vi "Add Rx Frames.vi"(8 "error in (no error)":errorcluster, 10 "CAN Frames":T1[](array[typedef]) {"payload" format="%x"; "timestamp" format="%<%.7X\n%x>T"; "type" items=["CAN Data"=0, "CAN Remote"=1, "CAN Bus Error"=2, "CAN 2.0 Data"=8, "CAN FD Data"=16, "CAN FD+BRS Data"=24, "J1939 Data"=192, "Delay"=224, "Log Trigger"=225, "Start Trigger"=226]; "identifier" format="%x"}, 11 "CANBus_Load_Calculator in":refnum<class "CANBus_Load_Calculator.lvclass">) -> (0 "error out":errorcluster, 3 "CANBus_Load_Calculator out":refnum<class "CANBus_Load_Calculator.lvclass">)   [LabVIEW 2018, in "NI-XNET Monitor Engine.lvlib" / "XNET-Bus-Load-Calculator.lvlib" / "CANBus_Load_Calculator.lvclass"]
uses:
  CANBus_Load_Calculator.lvclass
  <vilib>/xnet/xnet.llb/XNET Frame CAN.ctl
  <vilib>/xnet/xnet.llb/XNET Frame Type CAN.ctl
  CANBus_Load_Calculator.lvclass/CANBus_Load_Calculator.ctl
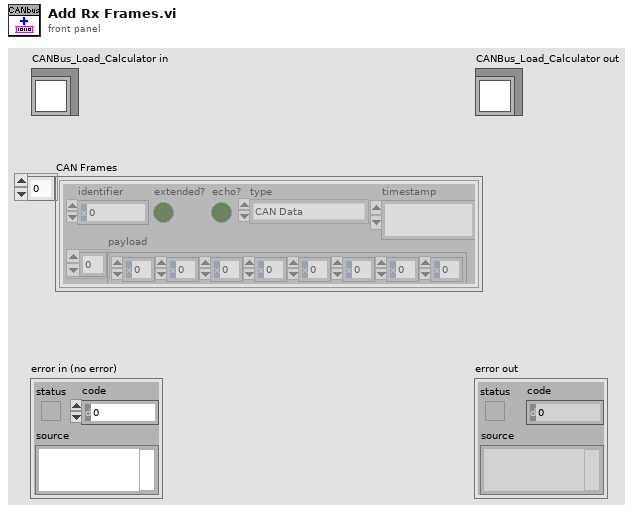
[diagram p1: front panel]
types:
  T1 = typedef "XNET Frame CAN.ctl" = cluster{"timestamp":timestamp, "payload":u8[], "identifier":u32, "type":T2, "extended?":bool, "echo?":bool}
  T2 = typedef "XNET Frame Type CAN.ctl" = u8
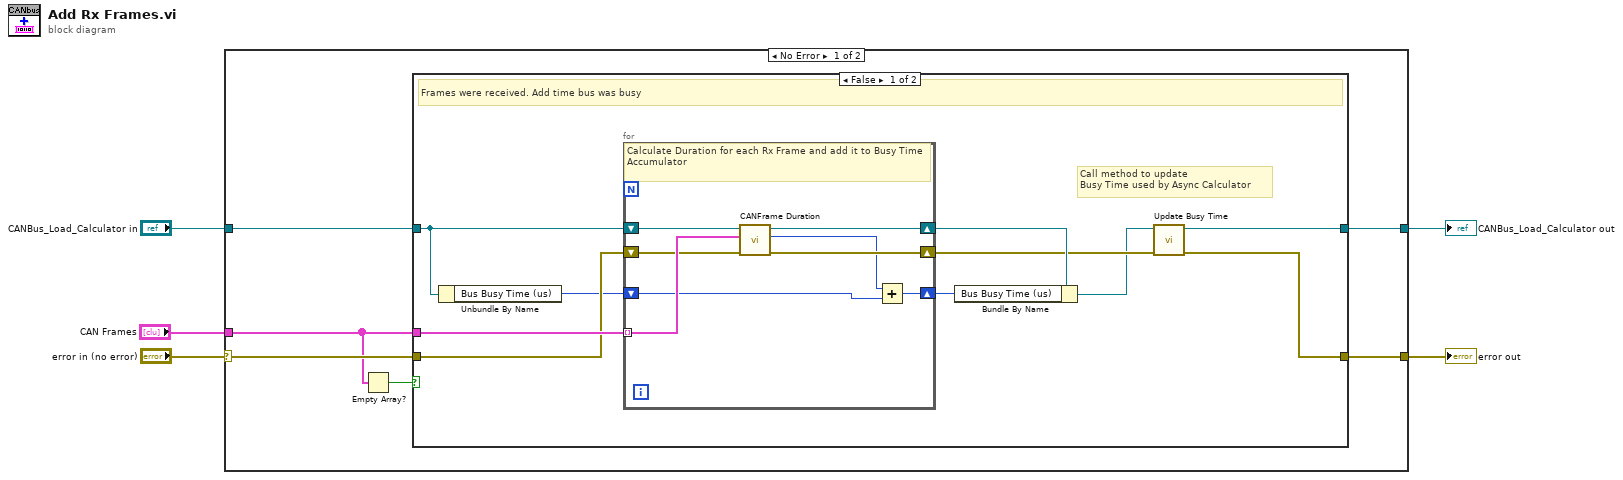
[diagram p0: block diagram]
diagram:
  n1 = case shown="No Error" "error in (no error)" {
    selector: "error in (no error)" -> [w11 w33]
    tunnel: [w8 w33] -> w4
    tunnel: [w9 w32] -> w2
    tunnel: "CANBus_Load_Calculator in" -> [w10 w32]
    tunnel: "CAN Frames" -> [w6 _]
    frame No Error {
      n2 = Empty Array?(array=w6) -> (empty?=w7:bool)
      n3 = case shown="False" w7 {
        tunnel: w11 -> [w20 w30]
        tunnel: w10 -> [w19 w31]
        tunnel: [w13 w31] -> w9
        tunnel: [w14 w30] -> w8
        tunnel: w6 -> [w21 _]
        frame False {
          # "Call method to update\nBusy Time used by Async Calculator"
          # "Frames were received. Add time bus was busy"
          n4 = Unbundle By Name(w19) -> ("Bus Busy Time (us)"=w18:u64)
          n5 = for {
            tunnel: w21 -> [w29] mode=indexing
            shift-right: [w28] -> w15
            shift-left: w20 -> [w27]
            shift-right: [w22] -> w16
            shift-left: w18 -> [w23]
            shift-right: [w26] -> w17
            shift-left: w19 -> [w25]
            # "Calculate Duration for each Rx Frame and add it to Busy Time Accumulator"
            n6 = call "CANFrame Duration.vi"("error in (no error)"=w27, "CAN frame"=w29, "CANBus_Load_Calculator in"=w25) -> ("error out"=w28:errorcluster, "Frame Duration (us)"=w24:u64, "CANBus_Load_Calculator out"=w26:refnum<class "CANBus_Load_Calculator.lvclass">)  [unwired: 6 in]
            n7 = Add(x=w24, y=w23) -> (x+y=w22:u64)
          }
          n8 = Bundle By Name(cluster=w17, "Bus Busy Time (us)"=w16) -> (w12:refnum<class "CANBus_Load_Calculator.lvclass">)
          n9 = call "Update Busy Time.vi"("error in (no error)"=w15, "GenBus_Load_Calculator in"=w12) -> ("error out"=w14:errorcluster, "GenBus_Load_Calculator out"=w13:refnum<class "CANBus_Load_Calculator.lvclass">)  [unwired: 8 in]
        }
        frame True {
          # "No new frames received. No action to take"
        }
      }
    }
    frame Error {
    }
  }
  "error out" <- w4
  "CANBus_Load_Calculator out" <- w2
